vi "Write Save Enable.vi"(8 "error in (no error)":errorcluster, 10 "Save Enable":bool, 11 "Generador in":refnum<class "Generador.lvclass">) -> (0 "error out":errorcluster, 3 "Generador out":refnum<class "Generador.lvclass">)   [LabVIEW 2020, in "Generador señal.lvlib" / "Generador.lvclass"]
uses:
  Generador.lvclass
  Generador.lvclass/Generador.ctl
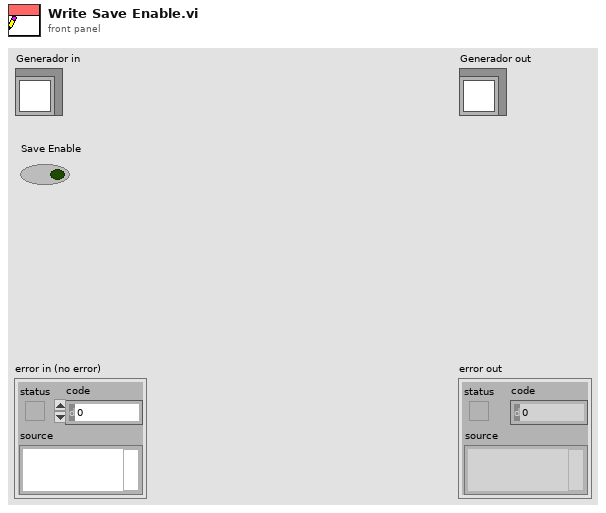
[diagram p1: front panel]
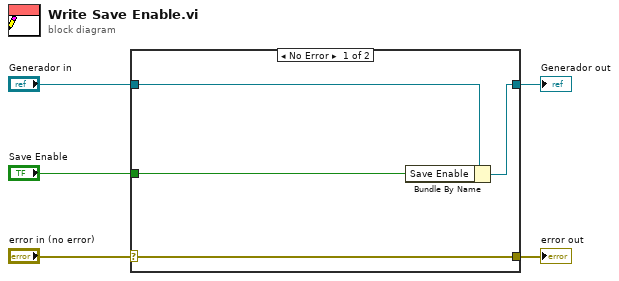
[diagram p0: block diagram]
diagram:
  n1 = case shown="No Error" "error in (no error)" {
    selector: "error in (no error)" -> [w9 w10]
    tunnel: [w9 w10] -> w4
    tunnel: [w7 w11] -> w2
    tunnel: "Generador in" -> [w8 w11]
    tunnel: "Save Enable" -> [w6 _]
    frame No Error {
      n2 = Bundle By Name(cluster=w8, "Save Enable"=w6) -> (w7:refnum<class "Generador.lvclass">)
    }
    frame Error {
    }
  }
  "error out" <- w4
  "Generador out" <- w2
